vi "MB Ethernet Example Slave MK2.vi"() -> ()   [LabVIEW 2012]
uses:
  API/Wrapper/API Main.lvlib
  API/Slave/Modbus Slave.lvclass
  API/Wrapper/Create TCP Slave.vi
  Data Model/Identification Parameters.ctl
  Data Model/Device Data Model.lvclass
  Master Function Definition/Read Device ID code.ctl
panel:
  in  "HR to write":u16[](array[numeric])=[1, 65535, 40000, 20000]
  in  "Set HR":bool
  in  "Set IR":bool
  in  "IR to write":u16[](array[numeric])=[1, 65535, 40000, 20000]
  in  "IR 6":u16
  in  "Set !":bool
  in  "! status":u8=1
  in  "Set Coils":bool
  in  "Set DI":bool
  in  "DI to write":bool[](array[boolean])=[FALSE, TRUE, FALSE, TRUE]
  in  "coils to write":bool[](array[boolean])=[FALSE, TRUE, FALSE, TRUE]
  in  "set objects":bool
  in  "Objects In":T1[](array[typedef])=[{"Object ID"=0, "Value"="National instruments"}, {"Object ID"=1, "Value"="42"}, {"Object ID"=2, "Value"="1.0.0"}] {"Object ID" format="%x"}
  in  "Coil 6":bool
  out "exception status":u8=1
  out "register values":u16[](array[numeric])=[1, 1, 65535, 40000, 20000, 6]
  out "discrete inputs":bool[](array[boolean])=[FALSE, FALSE, TRUE, FALSE, TRUE, TRUE]
  in  "Read Device ID code":T2
  out "Objects":T1[](array[typedef])=[{"Object ID"=0, "Value"="National instruments"}, {"Object ID"=1, "Value"="42"}, {"Object ID"=2, "Value"="1.0.0"}] {"Object ID" format="%x"}
  in  "Object Id":u8 format="%02x"
  out "holding reg":u16[](array[numeric])=[1, 1, 65535, 40000, 20000, 6]
  out "error out":errorcluster
  in  "stop":bool
  out "Coils":bool[](array[boolean])=[FALSE, FALSE, TRUE, FALSE, TRUE, TRUE] caption="Coils (Master can write coils)"
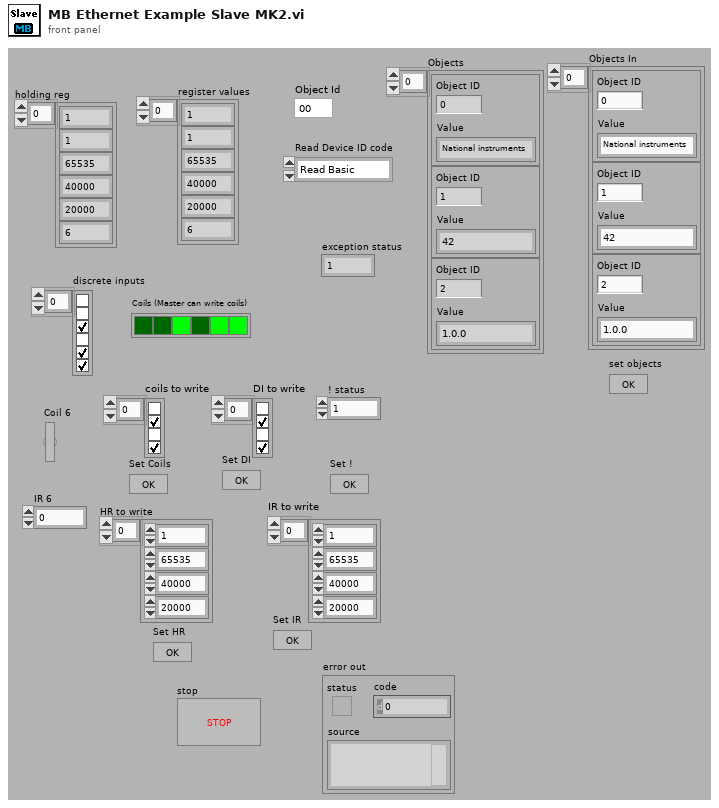
[diagram p1: front panel]
types:
  T1 = typedef "Device Data Model.lvclass/Identification Parameters.ctl" = cluster{"Object ID":u8, "Value":string}
  T2 = typedef "Device Data Model.lvclass/Read Device ID code.ctl" = enum8{"Read Basic", "Read Regular", "Read Extended", "Read Specific"}
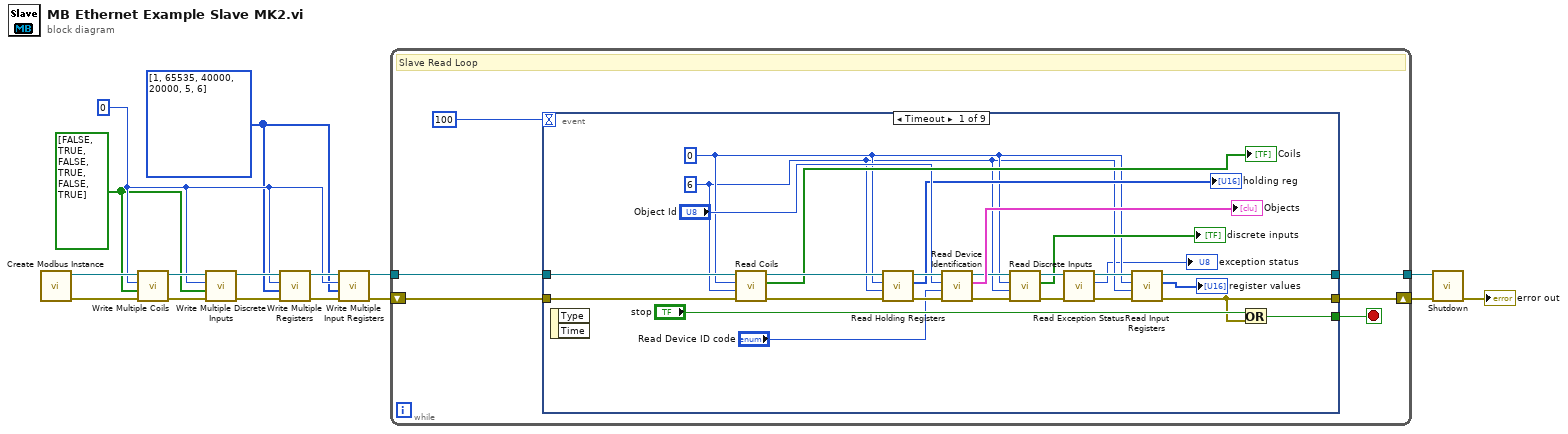
[diagram p0: block diagram]
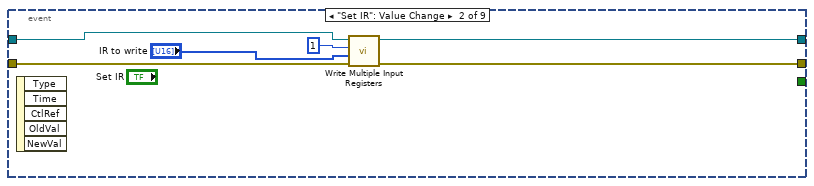
[diagram p2: hidden frame]
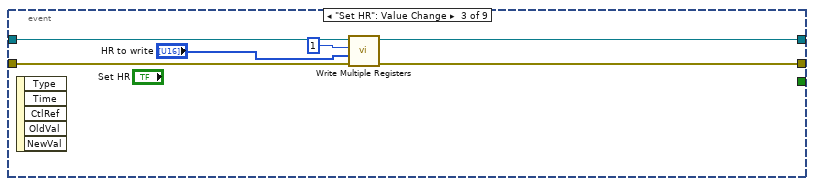
[diagram p3: hidden frame]
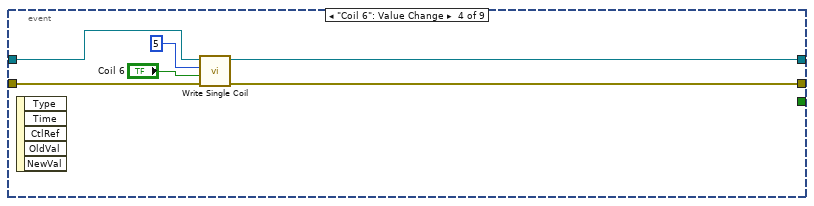
[diagram p4: hidden frame]
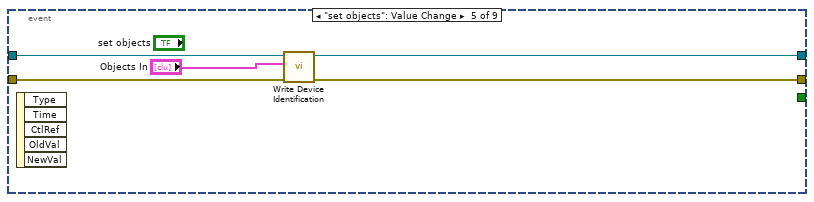
[diagram p5: hidden frame]
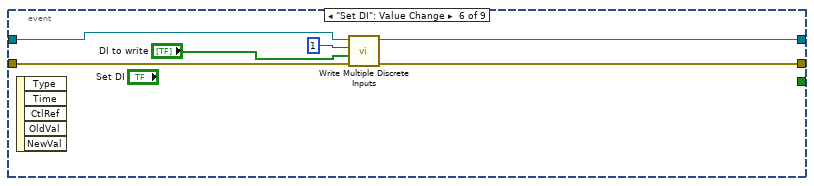
[diagram p6: hidden frame]
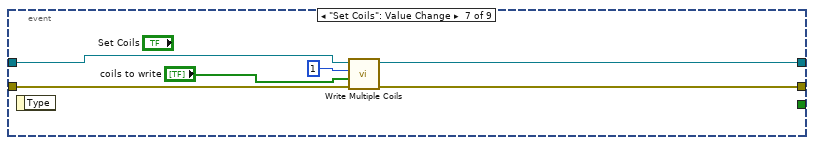
[diagram p7: hidden frame]
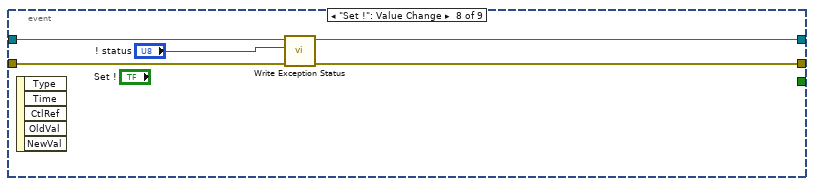
[diagram p8: hidden frame]
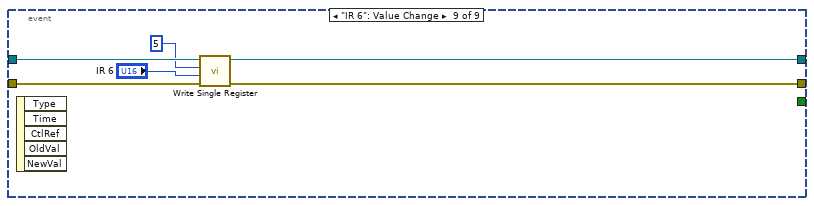
[diagram p9: hidden frame]
diagram:
  w1 = bool[] [FALSE, TRUE, FALSE, TRUE, FALSE, TRUE] ("coils to write")
  w2 = u16[] [1, 65535, 40000, 20000, 5, 6] ("registers")
  w3 = u16 0 ("starting address")
  n1 = call-poly "Create Modbus Instance.vi"() -> ("error out"=w7:errorcluster, "TCP slave instance"=w8:refnum<class "Modbus Slave.lvclass">)  [unwired: 10 in]
  n2 = call-dynamic "Write Multiple Coils.vi"("error in"=w7, "coils to write"=w1, "starting address"=w3, "Modbus slave in"=w8) -> ("error out"=w6:errorcluster, "Modbus slave out"=w9:refnum<class "Modbus Slave.lvclass">)  [unwired: 6 in]
  n3 = call-dynamic "Write Multiple Discrete Inputs.vi"("error in"=w6, "discrete inputs to write"=w1, "starting address"=w3, "Modbus slave in"=w9) -> ("error out"=w11:errorcluster, "Modbus slave out"=w10:refnum<class "Modbus Slave.lvclass">)  [unwired: 6 in]
  n4 = call-dynamic "Write Multiple Registers.vi"("error in"=w11, "registers to write"=w2, "starting address"=w3, "Modbus slave in"=w10) -> ("error out"=w12:errorcluster, "Modbus slave out"=w13:refnum<class "Modbus Slave.lvclass">)  [unwired: 6 in]
  n5 = call-dynamic "Write Multiple Input Registers.vi"("error in"=w12, "input registers to write"=w2, "starting address"=w3, "Modbus slave in"=w13) -> ("error out"=w5:errorcluster, "Modbus slave out"=w4:refnum<class "Modbus Slave.lvclass">)  [unwired: 6 in]
  n6 = while {
    tunnel: [w18] -> w16
    tunnel: w4 -> [w21]
    shift-right: [w19] -> w15
    shift-left: w5 -> [w20]
    stop <- w22 stop-if-true
    # "Slave Read Loop"
    n7 = event shown="[0] Timeout" {
      selector: _ -> [_ _ _ _ _ _ _ _ _]
      dyn-events: _ -> [_ _ _ _ _ _ _ _ _]
      timeout: 100 -> [_ _ _ _ _ _ _ _ _]
      tunnel: [w45 _ _ _ _ _ _ _ _] -> w22
      tunnel: w21 -> [w40 w51 w60 w63 w68 w77 w80 w87 w94]
      tunnel: w20 -> [w39 w52 w57 w64 w69 w76 w81 w88 w93]
      tunnel: [w35 w53 w58 w65 w70 w73 w82 w85 w92] -> w19
      tunnel: [w34 w54 w59 w66 w71 w72 w83 w84 w91] -> w18
      event Timeout {
        w25 = u16 6 ("Number of coils")
        w26 = u16 0 ("Starting Address")
        n8 = event-data() -> ()  [unwired: 1 in, 2 out]
        n9 = call-dynamic "Read Coils.vi"("error in"=w39, "number of inputs"=w25, "starting address"=w26, "Modbus slave in"=w40) -> ("error out"=w44:errorcluster, "coils"=→"Coils":bool[], "Modbus slave out"=w43:refnum<class "Modbus Slave.lvclass">)  [unwired: 5 in]
        n10 = call-dynamic "Read Holding Registers.vi"("error in"=w44, "number of inputs"=w25, "starting address"=w26, "Modbus slave in"=w43) -> ("error out"=w46:errorcluster, "register values"=→"holding reg":u16[], "Modbus slave out"=w47:refnum<class "Modbus Slave.lvclass">)  [unwired: 5 in]
        n11 = call-dynamic "Read Device Identification.vi"("error in"=w46, "read device ID code"="Read Device ID code", "object ID"="Object Id", "Modbus slave in"=w47) -> ("error out"=w31:errorcluster, "objects"=→"Objects":T1[], "Modbus slave out"=w28:refnum<class "Modbus Slave.lvclass">)  [unwired: 5 in]
        n12 = call-dynamic "Read Discrete Inputs.vi"("error in"=w31, "number of inputs"=w25, "starting address"=w26, "Modbus slave in"=w28) -> ("error out"=w32:errorcluster, "discrete inputs"=→"discrete inputs":bool[], "Modbus slave out"=w30:refnum<class "Modbus Slave.lvclass">)  [unwired: 5 in]
        n13 = call-dynamic "Read Exception Status.vi"("error in"=w32, "Modbus slave in"=w30) -> ("error out"=w33:errorcluster, "exception status"=→"exception status":u8, "Modbus slave out"=w29:refnum<class "Modbus Slave.lvclass">)  [unwired: 7 in]
        n14 = call-dynamic "Read Input Registers.vi"("error in"=w33, "number of inputs"=w25, "starting address"=w26, "Modbus slave in"=w29) -> ("error out"=w35:errorcluster, "register values"=→"register values":u16[], "Modbus slave out"=w34:refnum<class "Modbus Slave.lvclass">)  [unwired: 5 in]
        n15 = Or(x="stop", y=w35) -> (x .or. y?=w45:bool)
      }
      event "Set IR": Value Change {
        n16 = event-data() -> ()  [unwired: 1 in, 5 out]
        n17 = call-dynamic "Write Multiple Input Registers.vi"("error in"=w52, "input registers to write"="IR to write", "starting address"=u16 1, "Modbus slave in"=w51) -> ("error out"=w53:errorcluster, "Modbus slave out"=w54:refnum<class "Modbus Slave.lvclass">)  [unwired: 6 in]
      }
      event "Set HR": Value Change {
        n18 = event-data() -> ()  [unwired: 1 in, 5 out]
        n19 = call-dynamic "Write Multiple Registers.vi"("error in"=w57, "registers to write"="HR to write", "starting address"=u16 1, "Modbus slave in"=w60) -> ("error out"=w58:errorcluster, "Modbus slave out"=w59:refnum<class "Modbus Slave.lvclass">)  [unwired: 6 in]
      }
      event "Coil 6": Value Change {
        n20 = event-data() -> ()  [unwired: 1 in, 5 out]
        n21 = call-dynamic "Write Single Coil.vi"("error in"=w64, "coil to write"="Coil 6", "address"=u16 5, "Modbus slave in"=w63) -> ("error out"=w65:errorcluster, "Modbus slave out"=w66:refnum<class "Modbus Slave.lvclass">)  [unwired: 6 in]
      }
      event "set objects": Value Change {
        n22 = event-data() -> ()  [unwired: 1 in, 5 out]
        n23 = call-dynamic "Write Device Identification.vi"("error in"=w69, "objects"="Objects In", "Modbus slave in"=w68) -> ("error out"=w70:errorcluster, "Modbus slave out"=w71:refnum<class "Modbus Slave.lvclass">)  [unwired: 7 in]
      }
      event "Set DI": Value Change {
        n24 = event-data() -> ()  [unwired: 1 in, 5 out]
        n25 = call-dynamic "Write Multiple Discrete Inputs.vi"("error in"=w76, "discrete inputs to write"="DI to write", "starting address"=u16 1, "Modbus slave in"=w77) -> ("error out"=w73:errorcluster, "Modbus slave out"=w72:refnum<class "Modbus Slave.lvclass">)  [unwired: 6 in]
      }
      event "Set Coils": Value Change {
        n26 = event-data() -> ()  [unwired: 1 in, 1 out]
        n27 = call-dynamic "Write Multiple Coils.vi"("error in"=w81, "coils to write"="coils to write", "starting address"=u16 1, "Modbus slave in"=w80) -> ("error out"=w82:errorcluster, "Modbus slave out"=w83:refnum<class "Modbus Slave.lvclass">)  [unwired: 6 in]
      }
      event "Set !": Value Change {
        n28 = event-data() -> ()  [unwired: 1 in, 5 out]
        n29 = call "Write Exception Status.vi"("error in"=w88, "exception status"="! status", "Modbus slave in"=w87) -> ("error out"=w85:errorcluster, "Modbus slave out"=w84:refnum<class "Modbus Slave.lvclass">)  [unwired: 7 in]
      }
      event "IR 6": Value Change {
        n30 = event-data() -> ()  [unwired: 1 in, 5 out]
        n31 = call-dynamic "Write Single Register.vi"("error in"=w93, "register to write"="IR 6", "address"=u16 5, "Modbus slave in"=w94) -> ("error out"=w92:errorcluster, "Modbus slave out"=w91:refnum<class "Modbus Slave.lvclass">)  [unwired: 6 in]
      }
    }
  }
  n32 = call-dynamic "Shutdown.vi"("error in"=w15, "Modbus slave in"=w16) -> ("error out"=→"error out":errorcluster)  [unwired: 9 in]
